vi "Read DVR.vi"(8 "error in (no error)":errorcluster, 11 "Crosswinds in":refnum<class "Bubble.lvclass">) -> (0 "error out":errorcluster, 2 "DVR":refnum<data-value>, 3 "Crosswinds out":refnum<class "Bubble.lvclass">)   [LabVIEW 2020, in "Bubble.lvclass"]
uses:
  Bubble.lvclass
  DVR Cluster.ctl
  Spot Cluster.ctl
  State Enum.ctl
  Role Enum.ctl
  Bubble.lvclass/Bubble.ctl
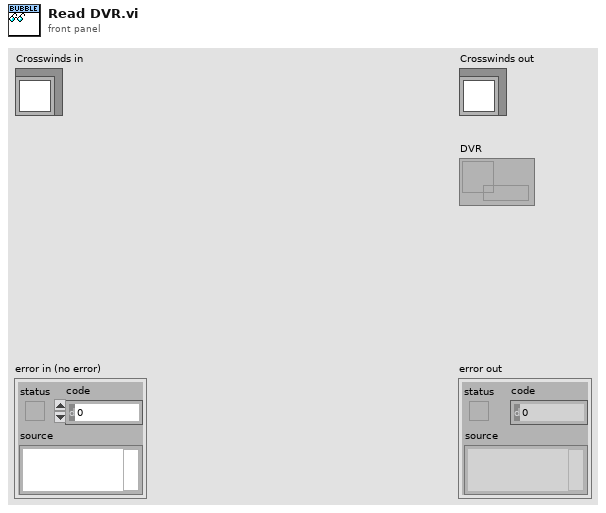
[diagram p1: front panel]
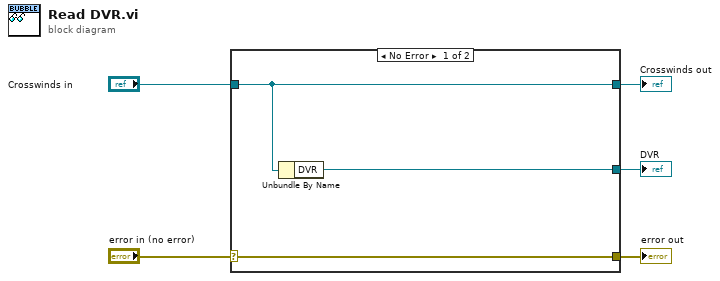
[diagram p0: block diagram]
diagram:
  n1 = case shown="No Error" "error in (no error)" {
    selector: "error in (no error)" -> [w8 w9]
    tunnel: [w8 w9] -> w4
    tunnel: [w7 w10] -> w2
    tunnel: "Crosswinds in" -> [w7 w10]
    tunnel: [w6 _] -> w1
    frame No Error {
      n2 = Unbundle By Name(w7) -> ("DVR"=w6:refnum<data-value>)
    }
    frame Error {
    }
  }
  "error out" <- w4
  "Crosswinds out" <- w2
  "DVR" <- w1
